vi "init_CV.vi"(3 "input_machine_reference.lvclass":refnum<class "machine.lvclass">) -> (0 "output_CV_parameters":T1, 1 "output_machine_reference.lvclass":refnum<class "machine.lvclass">)   [LabVIEW 2014, in "technique_parameters.lvclass"]
uses:
  technique_parameters.lvclass
  machine_ops/machine.lvclass
panel:
  in  "Exit":bool
  in  "Set":bool
  in  "Negative Direction?":bool
  in  "Sense Range":T2(ring)
  in  "Cycles":i32=1 min=1 max=30
  in  "End Voltage Level":dbl min=-10.0 max=10.0
  in  "Step Time":i32=20 min=1 max=50
  in  "Voltage per sec":dbl=1e-05 min=1e-05 max=1.0
  in  "Low Voltage Limit":dbl min=-10.0 max=10.0
  in  "High Voltage Limit":dbl min=-10.0 max=10.0
  in  "Initial Voltage Level":dbl=-10.0 min=-10.0 max=-10.0
  # "V / s"
  # "V"
  # "V"
  # "step / s"
  # "V"
  # "V"
  # "A"
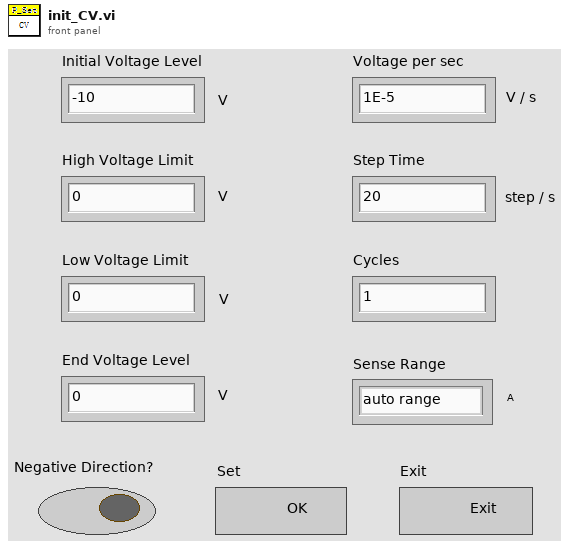
[diagram p1: front panel]
types:
  T1 = cluster{"init_volt":dbl, "high_volt":dbl, "low_volt":dbl, "end_volt":dbl, "volt_per_sec":dbl, "step_time":i32, "cycles":i32, "sense_range":enum16{"auto range", "1E-1", "1E-2", "1E-3", "1E-4", "1E-5", "1E-6", "1E-7", "1E-8", "1E-9"}, "is_negative":bool}
  T2 = enum16{"auto range", "1E-1", "1E-2", "1E-3", "1E-4", "1E-5", "1E-6", "1E-7", "1E-8", "1E-9"}
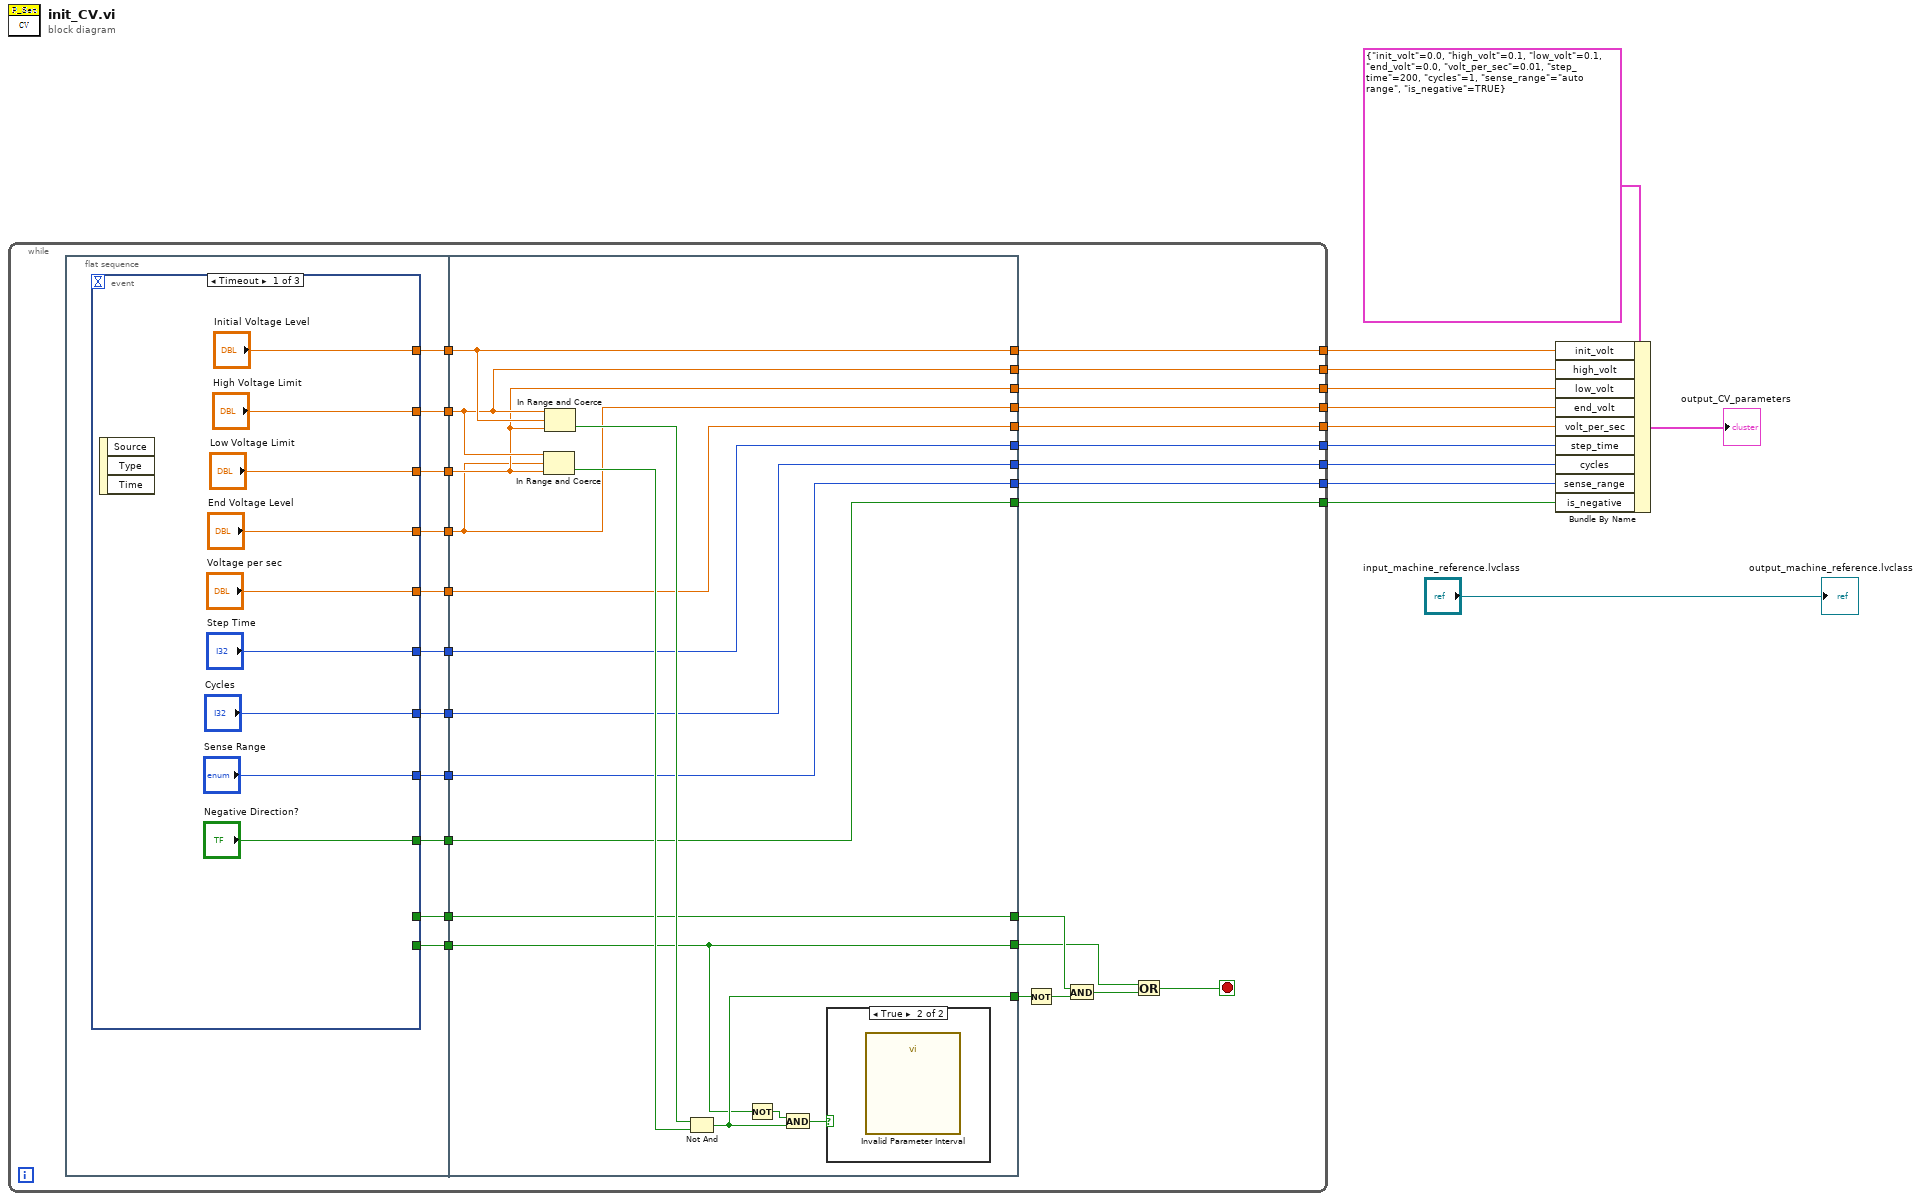
[diagram p0: block diagram]
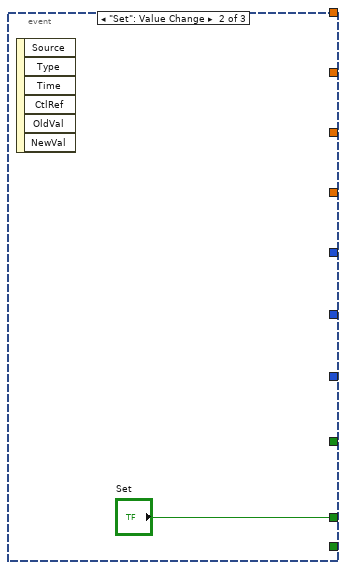
[diagram p2: hidden frame]
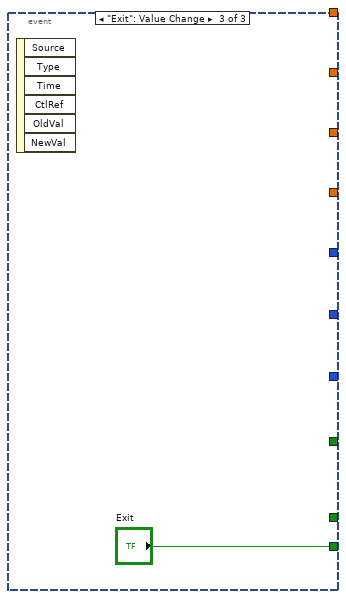
[diagram p3: hidden frame]
diagram:
  n1 = while {
    tunnel: [w25] -> w11
    tunnel: [w24] -> w10
    tunnel: [w23] -> w9
    tunnel: [w22] -> w8
    tunnel: [w21] -> w7
    tunnel: [w20] -> w6
    tunnel: [w19] -> w5
    tunnel: [w18] -> w4
    tunnel: [w17] -> w3
    stop <- w14 stop-if-true
    n2 = flat-sequence {
      tunnel: [w49] -> w38
      tunnel: [w48] -> w37
      tunnel: [w47] -> w36
      tunnel: [w46] -> w35
      tunnel: [w45] -> w34
      tunnel: [w44] -> w33
      tunnel: [w43] -> w32
      tunnel: [w42] -> w31
      tunnel: [w41] -> w30
      tunnel: [w40] -> w29
      tunnel: [w39] -> w28
      tunnel: w38 -> [w65]
      tunnel: w37 -> [w66]
      tunnel: w36 -> [w67]
      tunnel: w35 -> [w68]
      tunnel: w34 -> [w69]
      tunnel: w33 -> [w70]
      tunnel: w32 -> [w71]
      tunnel: w31 -> [w72]
      tunnel: w30 -> [w73]
      tunnel: [w63] -> w27
      tunnel: [w74] -> w16
      tunnel: w29 -> [w74]
      tunnel: [w61] -> w13
      tunnel: w28 -> [w61]
      tunnel: [w73] -> w25
      tunnel: [w72] -> w24
      tunnel: [w71] -> w23
      tunnel: [w70] -> w22
      tunnel: [w69] -> w21
      tunnel: [w68] -> w20
      tunnel: [w67] -> w19
      tunnel: [w66] -> w18
      tunnel: [w65] -> w17
      frame #0 {
        n3 = event shown="[0] Timeout" {
          selector: _ -> [_ _ _]
          dyn-events: _ -> [_ _ _]
          timeout: _ -> [_ _ _]
          tunnel: [_ "Set" _] -> w40
          tunnel: [_ _ "Exit"] -> w39
          tunnel: ["Negative Direction?" _ _] -> w49
          tunnel: ["Sense Range" _ _] -> w48
          tunnel: ["Cycles" _ _] -> w47
          tunnel: ["Step Time" _ _] -> w46
          tunnel: ["Voltage per sec" _ _] -> w45
          tunnel: ["End Voltage Level" _ _] -> w44
          tunnel: ["Low Voltage Limit" _ _] -> w43
          tunnel: ["High Voltage Limit" _ _] -> w42
          tunnel: ["Initial Voltage Level" _ _] -> w41
          event Timeout {
            n4 = event-data() -> ()  [unwired: 1 in, 3 out]
          }
          event "Set": Value Change {
            n5 = event-data() -> ()  [unwired: 1 in, 6 out]
          }
          event "Exit": Value Change {
            n6 = event-data() -> ()  [unwired: 1 in, 6 out]
          }
        }
      }
      frame #1 {
        n7 = In Range and Coerce(upper limit=w72, x=w70, lower limit=w71) -> (In Range?=w75:bool)  [unwired: 1 out]
        n8 = In Range and Coerce(upper limit=w72, x=w73, lower limit=w71) -> (In Range?=w76:bool)  [unwired: 1 out]
        n9 = Not And(1:w75, 2:w76) -> (0:w63:bool)
        n10 = Not(x=w61) -> (.not. x?=w62:bool)
        n11 = And(x=w62, y=w63) -> (x .and. y?=w64:bool)
        n12 = case shown="True" w64 {
          frame False {
          }
          frame True {
            n13 = call "Invalid Parameter Interval"() -> ()  [unwired: 10 in, 2 out]
          }
        }
      }
    }
    n14 = Not(x=w27) -> (.not. x?=w26:bool)
    n15 = And(x=w16, y=w26) -> (x .and. y?=w15:bool)
    n16 = Or(x=w13, y=w15) -> (x .or. y?=w14:bool)
  }
  n17 = Bundle By Name(cluster=T1 {"init_volt"=0.0, "high_volt"=0.1, "low_volt"=0.1, "end_volt"=0.0, "volt_per_sec"=0.01, "step_time"=200, "cycles"=1, "sense_range"=enum."auto range", "is_negative"=TRUE}, "init_volt"=w11, "high_volt"=w10, "low_volt"=w9, "end_volt"=w8, "volt_per_sec"=w7, "step_time"=w6, "cycles"=w5, "sense_range"=w4, "is_negative"=w3) -> (→"output_CV_parameters":T1)
  "output_machine_reference.lvclass" <- "input_machine_reference.lvclass"
